vi "Configure OVP.vi"(7 "Enable OVP (T: Enable)":bool=TRUE, 8 "error in (no error)":errorcluster, 9 "Voltage Limit (6.5 V)":dbl=6.5 format="%.2f", 10 "Channel (0: 30V Channel)":T1 caption="Channel (0: +6V)" items=["30V/3A Channel", "30V/3A Channel", "5V/3A Channel"], 11 "VISA resource name":refnum<visa-resource-name>) -> (0 "error out":errorcluster, 3 "VISA resource name out":refnum<visa-resource-name>)   [LabVIEW 2020, in "Library Instrument & Equipement.lvlib" / "Library Power_Supply.lvlib" / "RIGOL DP800 Series.lvlib"]
doc: "Configures over voltage protection (OVP) of the power supply. Specify the voltage limit and whether to enable or disable OVP."
uses:
  RIGOL DP800 Series.lvlib
  Channels.ctl
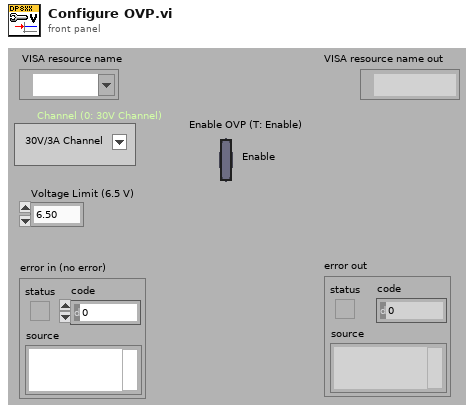
[diagram p1: front panel]
types:
  T1 = typedef "Library Instrument & Equipement.lvlib/Library Power_Supply.lvlib/RIGOL DP800 Series.lvlib/Channels.ctl" = i32
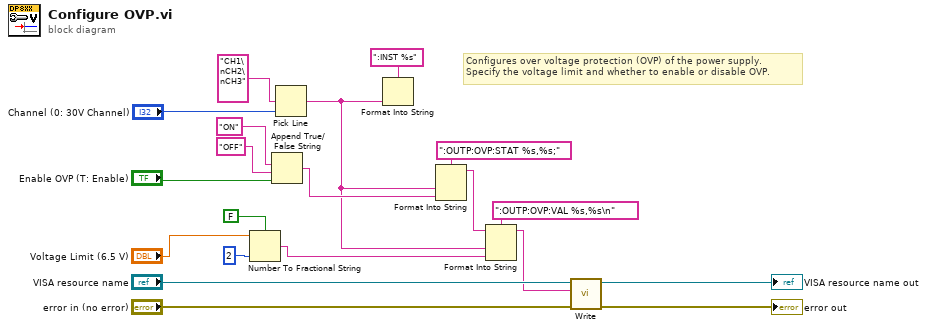
[diagram p0: block diagram]
diagram:
  # "Configures over voltage protection (OVP) of the power supply.  \nSpecify the voltage limit and whether to enable or disable OVP."
  n1 = Number To Fractional String(use system decimal point (T)=FALSE ("utiliser le séparateur décimal du système (V)"), number="Voltage Limit (6.5 V)", precision (6)=i16 2 ("précision (6)")) -> (F-format string=w1:string)  [unwired: 1 in]
  n2 = Append True/False String(1:"Enable OVP (T: Enable)", 2:"OFF", 3:"ON") -> (0:w15:string)  [unwired: 1 out]
  n3 = Pick Line(multi-line string="CH1\nCH2\nCH3", line index="Channel (0: 30V Channel)") -> (output string=w11:string)  [unwired: 1 out]
  n4 = Format Into String(format string=":INST %s", w11) -> ()  [unwired: 2 in, 2 out]
  n5 = Format Into String(format string=":OUTP:OVP:STAT %s,%s;", w11, w15) -> (resulting string=w14:string)  [unwired: 2 in, 1 out]
  n6 = Format Into String(format string=":OUTP:OVP:VAL %s,%s\n", initial string=w14, w11, w1) -> (resulting string=w6:string)  [unwired: 1 in, 1 out]
  n7 = call "Write.vi"("error in (no error)"="error in (no error)", "Write Buffer (\"\")"=w6, "VISA resource name"="VISA resource name") -> ("error out"=→"error out":errorcluster, "VISA resource name out"=→"VISA resource name out":refnum<visa-resource-name>)  [unwired: 7 in]
